vi "Fast Cash MSG.vi"(8 "error in":errorcluster, 11 "ATM Data":T1={"UI Refs"={"Right Buttons"=refnum, "Left Buttons"=refnum, "User Input"=refnum, "ATM Messages"=refnum, "Left Menu"=refnum, "Right Menu"=refnum, "Enter"=refnum}, "Map"={}, "Login Valid?"=FALSE, "Queue Message"=refnum, "State"=enum."None", "User"={"Pin"="", "First Name"="", "Last Name"="", "Balance"=0.0, "Login Valid?"=FALSE}, "Main States"={"Message"="Initialize", "Data"=variant}}) -> (0 "error out":errorcluster, 3 "ATM Data Out":T1={"UI Refs"={"Right Buttons"=refnum, "Left Buttons"=refnum, "User Input"=refnum, "ATM Messages"=refnum, "Left Menu"=refnum, "Right Menu"=refnum, "Enter"=refnum}, "Map"={}, "Login Valid?"=FALSE, "Queue Message"=refnum, "State"=enum."None", "User"={"Pin"="", "First Name"="", "Last Name"="", "Balance"=0.0, "Login Valid?"=FALSE}, "Main States"={"Message"="Initialize", "Data"=variant}})   [LabVIEW 2020, in "ATM Machine.lvlib"]
uses:
  ATM Machine.lvlib
  Cluster - ATM Machine Data.ctl
  Users/khemr/OneDrive/Desktop/Labview Training/CLD/New ATM_KR/ATM Machine/Cluster - Message Cluster.ctl
  Enum - ATM States.ctl
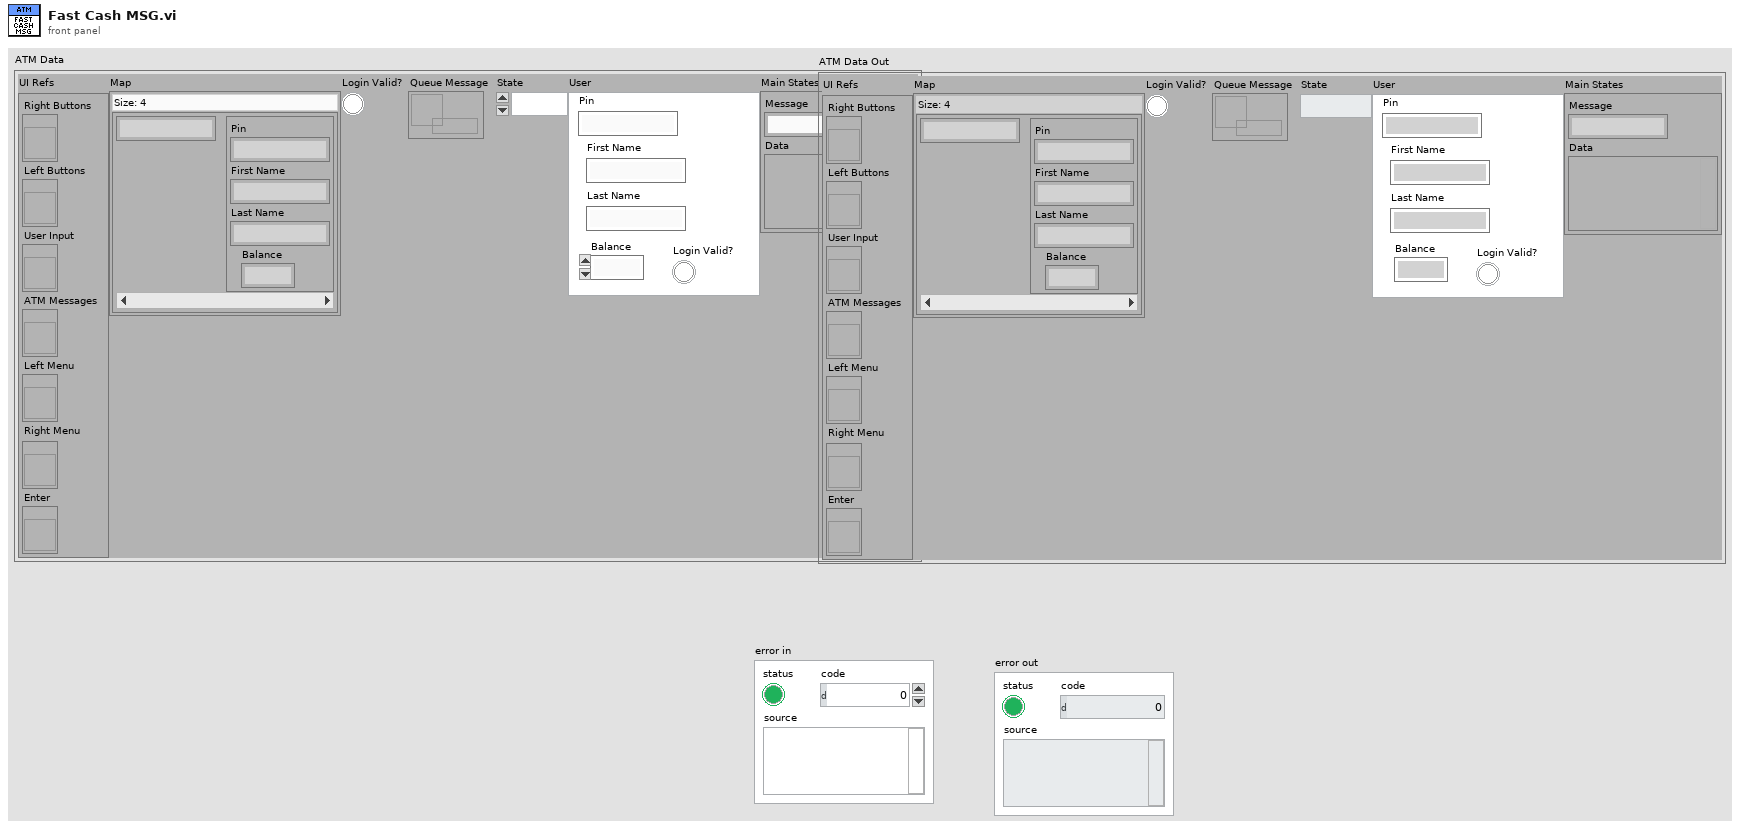
[diagram p1: front panel]
types:
  T1 = typedef "ATM Machine.lvlib/Cluster - ATM Machine Data.ctl" = cluster{"UI Refs":cluster{"Right Buttons":refnum<vi>, "Left Buttons":refnum<vi>, "User Input":refnum<vi>, "ATM Messages":refnum<vi>, "Left Menu":refnum<vi>, "Right Menu":refnum<vi>, "Enter":refnum<vi>}, "Map":map{string, cluster{"Pin":string, "First Name":string, "Last Name":string, "Balance":dbl}}, "Login Valid?":bool, "Queue Message":refnum<queue>, "State":T2, "User":cluster{"Pin":string, "First Name":string, "Last Name":string, "Balance":dbl, "Login Valid?":bool}, "Main States":cluster{"Message":string, "Data":variant}}
  T2 = typedef "ATM Machine.lvlib/Enum - ATM States.ctl" = enum16{"None", "Deposit", "Withdraw", "Card Inserted", "Balance Inquiry", "Return Card and Terminate", "Fast Cash"}
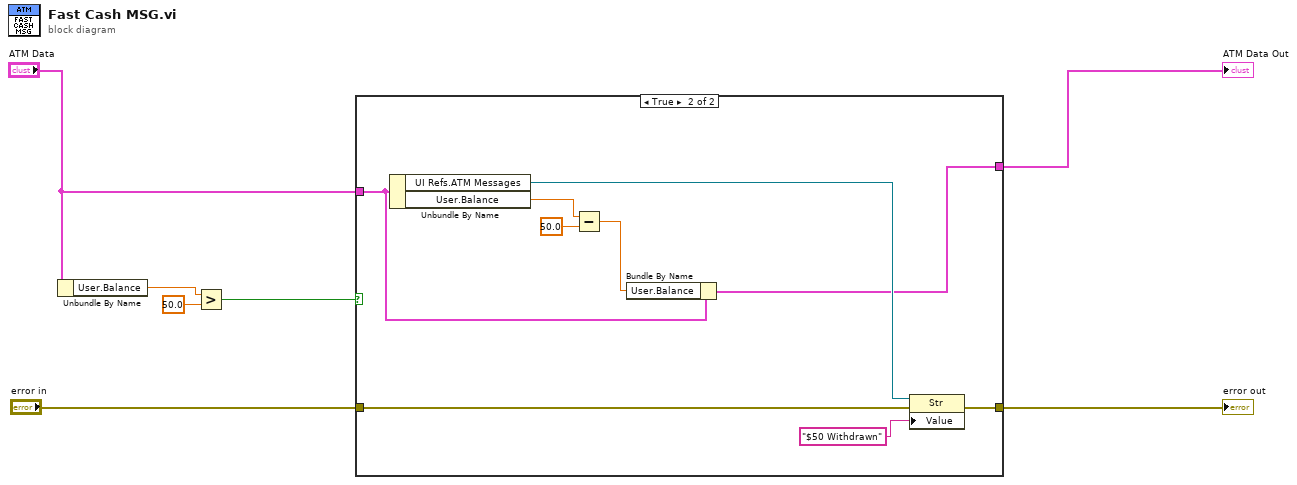
[diagram p0: block diagram]
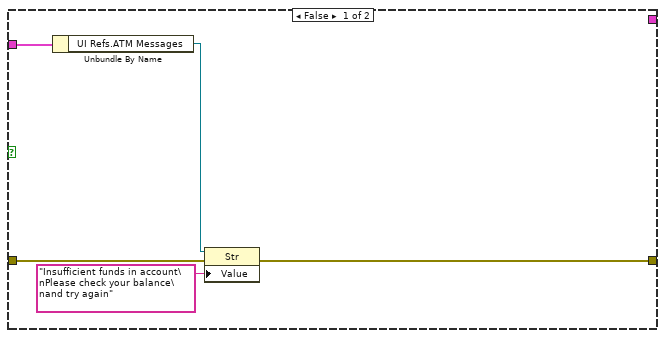
[diagram p2: hidden frame]
diagram:
  n1 = Unbundle By Name("ATM Data") -> ("User.Balance"=w7:dbl)
  n2 = Greater?(x=w7, y=50.0) -> (0:w3:bool)
  n3 = case shown="True" w3 {
    tunnel: [w10 w21] -> w5
    tunnel: "error in" -> [w11 w20]
    tunnel: "ATM Data" -> [w12 w15]
    tunnel: [_ w14] -> w1
    frame False {
      n4 = Unbundle By Name(w12) -> ("UI Refs.ATM Messages"=w9:refnum<vi>)
      n5 = property class="Str"(reference=w9, error in=w11, "Value"="Insufficient funds in account\nPlease check your balance\nand try again") -> (error out=w10:errorcluster)  [unwired: 1 out]
    }
    frame True {
      n6 = Unbundle By Name(w15) -> ("UI Refs.ATM Messages"=w19:refnum<vi>, "User.Balance"=w17:dbl)
      n7 = Subtract(x=w17, y=50.0) -> (x-y=w13:dbl)
      n8 = Bundle By Name(cluster=w15, "User.Balance"=w13) -> (w14:T1)
      n9 = property class="Str"(reference=w19, error in=w20, "Value"="$50 Withdrawn") -> (error out=w21:errorcluster)  [unwired: 1 out]
    }
  }
  "ATM Data Out" <- w1
  "error out" <- w5
